vi "Triangle scan Sub VI vertical.vi"(6 "X End  (um)":dbl, 8 "Handle In":i32, 9 "X Start  (um)":dbl, 10 "Y End  (um)":dbl, 11 "Y Start  (um)":dbl) -> (2 "X Position (um) 2":dbl(graph), 3 "Y Position (um) 2":dbl(graph))   [LabVIEW 2019]
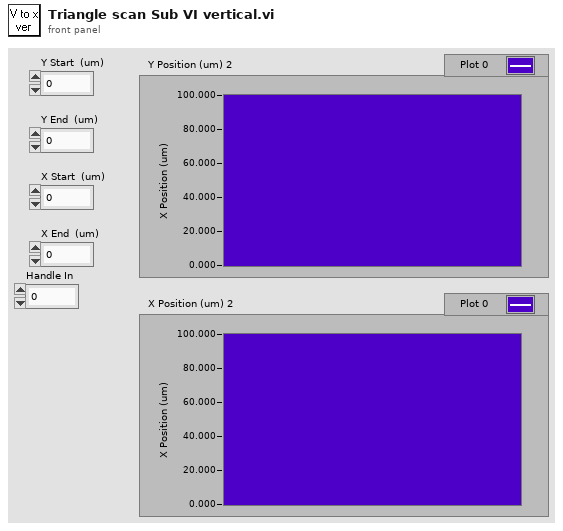
[diagram p1: front panel]
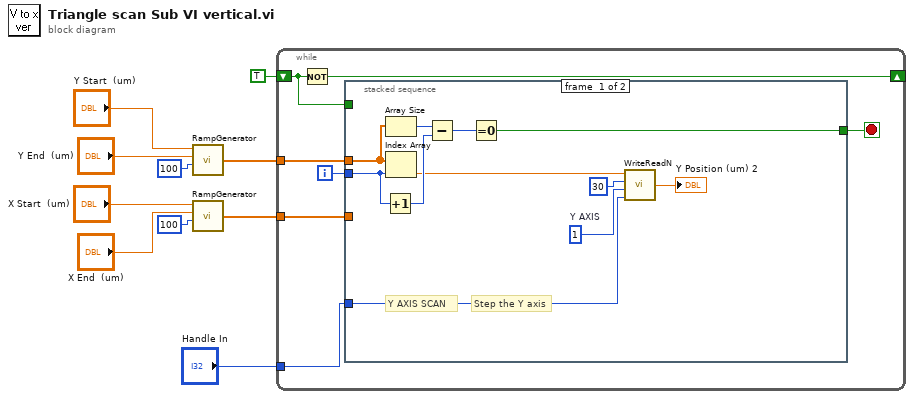
[diagram p0: block diagram]
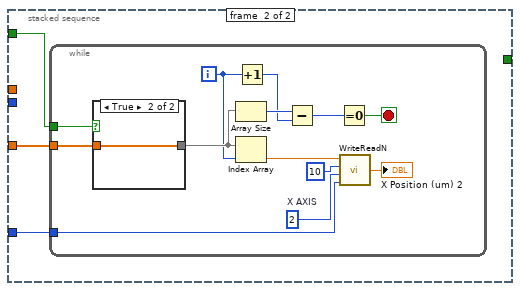
[diagram p2: hidden frame]
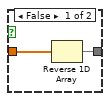
[diagram p3: hidden frame]
diagram:
  n1 = call "RampGenerator.vi"("Number of Positions"=u16 100 ("Y Samples"), "End  (um)"="Y End  (um)", "Start  (um)"="Y Start  (um)") -> ("Array"=w10:dbl[])  [unwired: 1 in]
  n2 = call "RampGenerator.vi"("Number of Positions"=u16 100 ("X Samples"), "End  (um)"="X End  (um)", "Start  (um)"="X Start  (um)") -> ("Array"=w2:dbl[])  [unwired: 1 in]
  n3 = while {
    tunnel: w2 -> [w15]
    tunnel: w10 -> [w12]
    shift-right: [w13] -> _
    shift-left: TRUE -> [w14]
    tunnel: "Handle In" -> [w11]
    i -> [w16]
    stop <- w17 stop-if-true
    n4 = Not(x=w14) -> (.not. x?=w13:bool)
    n5 = stacked-sequence {
      tunnel: w12 -> [w27 _]
      tunnel: [w25 _] -> w17
      tunnel: w16 -> [w24 _]
      tunnel: w15 -> [_ w31]
      tunnel: w14 -> [_ w30]
      tunnel: w11 -> [w18 w29]
      frame #0 {
        w19 = 1  # Y AXIS
        # "Step the Y axis"
        # "Y AXIS SCAN"
        n6 = Increment(x=w24) -> (x+1=w23:i32)
        n7 = Array Size(array=w27) -> (size(s)=w26:i32)
        n8 = Index Array(array=w27, index=w24) -> (element=w21:dbl)
        n9 = Subtract(x=w26, y=w23) -> (x-y=w28:i32)
        n10 = Equal To 0?(x=w28) -> (x = 0?=w25:bool)
        n11 = call "WriteReadN.vi"("Handle"=w18, "Axis"=w19, "Delay (ms)"=u32 30 ("Y DELAY (ms)"), "Move to (um)"=w21) -> ("Current Position (um)"=→"Y Position (um) 2":dbl)
      }
      frame #1 {
        n12 = while {
          tunnel: w31 -> [w43]
          tunnel: w30 -> [w41]
          tunnel: w29 -> [w35]
          i -> [w36]
          stop <- w39 stop-if-true
          w32 = 2  # X AXIS
          n13 = case shown="True" w41 {
            tunnel: w43 -> [w45 w47]
            tunnel: [w46 w47] -> w42
            frame False {
              n14 = Reverse 1D Array(array=w45) -> (reversed array=w46:dbl[])
            }
            frame True {
            }
          }
          n15 = Array Size(array=w42) -> (size(s)=w40:i32)
          n16 = Index Array(array=w42, index=w36) -> (element=w34:dbl)
          n17 = Increment(x=w36) -> (x+1=w37:i32)
          n18 = Subtract(x=w40, y=w37) -> (x-y=w44:i32)
          n19 = Equal To 0?(x=w44) -> (x = 0?=w39:bool)
          n20 = call "WriteReadN.vi"("Handle"=w35, "Axis"=w32, "Delay (ms)"=u32 10 ("X DELAY (ms)"), "Move to (um)"=w34) -> ("Current Position (um)"=→"X Position (um) 2":dbl)
        }
      }
    }
  }
